vi "PLC.SendReasembly.vi"(8 "error in":errorcluster, 10 "Reasembly data":T11, 11 "Data_in":T1={"Status"={"Idx"=0, "ConnRef"=0, "State"=enum."Off", "LiveBitTimer"=timestamp(0 s since 1904-01-01)}, "Sets"={"Enable"=FALSE, "IP"="", "Rack"=0, "Slot"=0, "LifeBitTimer_s"=0.0, "DataBlockAddr_PCStatus"=0, "DataBlockAddr_PLCStatus"=1, "DataBlockAddr_PLCNewData"=[], "DataBlockSize_PLCNewData"=[], "DataBlockAddr_PLCChangeOver"=[], "DataBlockSize_PLCChangeOver"=[], "DataBlockAddr_PCChangeOver"=[], "DataBlockAddr_PLCCheckStatus"=[], "DataBlockSize_PLCCheckStatus"=[], "DataBlockAddr_PCCheckStatus"=[]}, "PCstatus"={"General"={"LifeBit"=FALSE, "DbRun"=FALSE}, "Stations"=[]}, "PLCstatus"={"General"={"LifeBit"=FALSE}, "Stations"=[]}}) -> (0 "error out":errorcluster, 2 "PlcConfirmation":T11, 3 "Data out":T1={"Status"={"Idx"=0, "ConnRef"=0, "State"=enum."Off", "LiveBitTimer"=timestamp(0 s since 1904-01-01)}, "Sets"={"Enable"=FALSE, "IP"="", "Rack"=0, "Slot"=0, "LifeBitTimer_s"=0.0, "DataBlockAddr_PCStatus"=0, "DataBlockAddr_PLCStatus"=1, "DataBlockAddr_PLCNewData"=[], "DataBlockSize_PLCNewData"=[], "DataBlockAddr_PLCChangeOver"=[], "DataBlockSize_PLCChangeOver"=[], "DataBlockAddr_PCChangeOver"=[], "DataBlockAddr_PLCCheckStatus"=[], "DataBlockSize_PLCCheckStatus"=[], "DataBlockAddr_PCCheckStatus"=[]}, "PCstatus"={"General"={"LifeBit"=FALSE, "DbRun"=FALSE}, "Stations"=[]}, "PLCstatus"={"General"={"LifeBit"=FALSE}, "Stations"=[]}})   [LabVIEW 2016]
uses:
  PLC.CheckStatusReassembly.ctl
  PLC.Data.ctl
  PLC.Data.Status.ctl
  PLC.State.ctl
  PLC.Data.Sets.ctl
  LowLevel/PLC.DataBlock.PCstatus.ctl
  LowLevel/PLC.DataBlock.PCstatus.General.ctl
  LowLevel/PLC.DataBlock.PCstatus.Station.ctl
  LowLevel/PLC.DataBlock.PLCstatus.ctl
  LowLevel/PLC.DataBlock.PLCstatus.General.ctl
  LowLevel/PLC.DataBlock.PLCstatus.Station.ctl
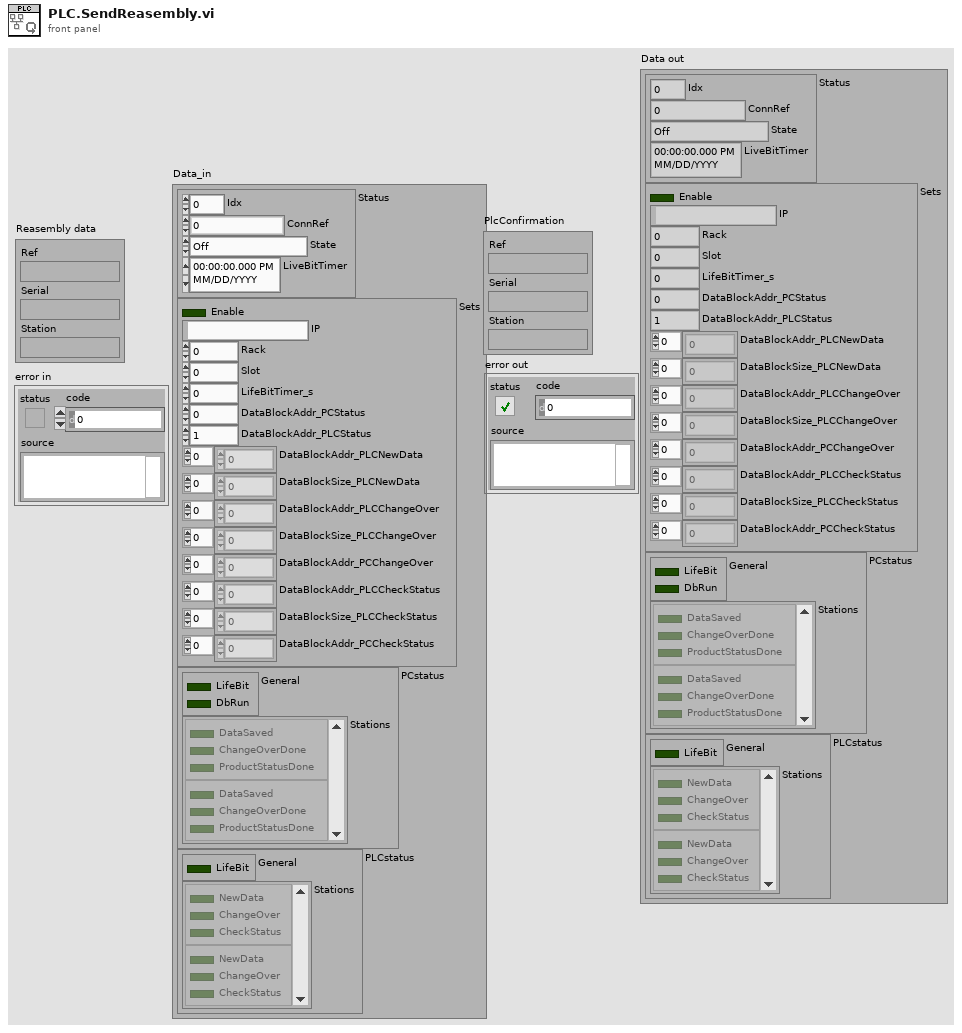
[diagram p1: front panel]
types:
  T1 = typedef "PLC.Data.ctl" = cluster{"Status":T2, "Sets":T4, "PCstatus":T5, "PLCstatus":T8}
  T2 = typedef "PLC.Data.Status.ctl" = cluster{"Idx":i32, "ConnRef":u64, "State":T3, "LiveBitTimer":timestamp}
  T3 = typedef "PLC.State.ctl" = enum32{"Off", "Error", "Idle", "Run"}
  T4 = typedef "PLC.Data.Sets.ctl" = cluster{"Enable":bool, "IP":string, "Rack":i32, "Slot":i32, "LifeBitTimer_s":dbl, "DataBlockAddr_PCStatus":i32, "DataBlockAddr_PLCStatus":i32, "DataBlockAddr_PLCNewData":i32[], "DataBlockSize_PLCNewData":i32[], "DataBlockAddr_PLCChangeOver":i32[], "DataBlockSize_PLCChangeOver":i32[], "DataBlockAddr_PCChangeOver":i32[], "DataBlockAddr_PLCCheckStatus":i32[], "DataBlockSize_PLCCheckStatus":i32[], "DataBlockAddr_PCCheckStatus":i32[]}
  T5 = typedef "PLC.DataBlock.PCstatus.ctl" = cluster{"General":T6, "Stations":T7[]}
  T6 = typedef "PLC.DataBlock.PCstatus.General.ctl" = cluster{"LifeBit":bool, "DbRun":bool}
  T7 = typedef "PLC.DataBlock.PCstatus.Station.ctl" = cluster{"DataSaved":bool, "ChangeOverDone":bool, "ProductStatusDone":bool}
  T8 = typedef "PLC.DataBlock.PLCstatus.ctl" = cluster{"General":T9, "Stations":T10[]}
  T9 = typedef "PLC.DataBlock.PLCstatus.General.ctl" = cluster{"LifeBit":bool}
  T10 = typedef "PLC.DataBlock.PLCstatus.Station.ctl" = cluster{"NewData":bool, "ChangeOver":bool, "CheckStatus":bool}
  T11 = typedef "PLC.CheckStatusReassembly.ctl" = cluster{"Ref":string, "Serial":string, "Station":string}
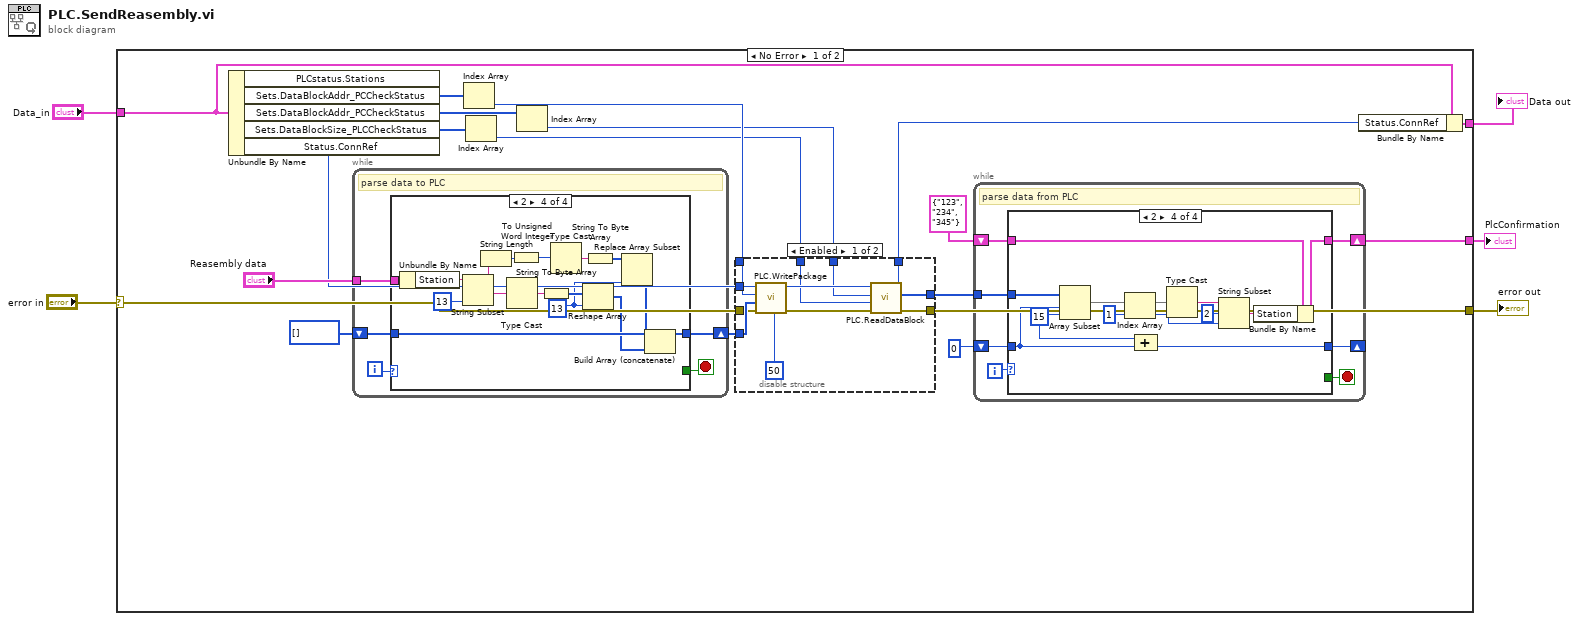
[diagram p0: block diagram]
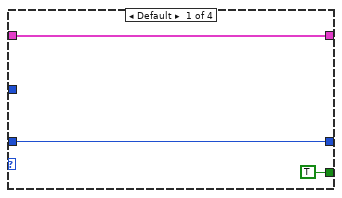
[diagram p3: hidden frame]
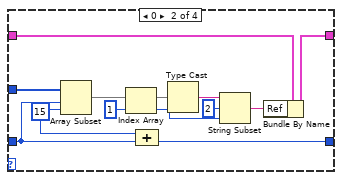
[diagram p4: hidden frame]
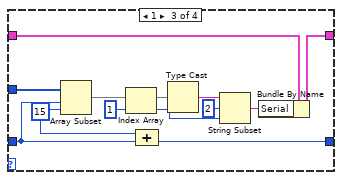
[diagram p5: hidden frame]
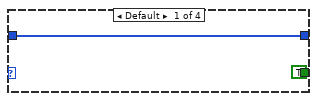
[diagram p6: hidden frame]
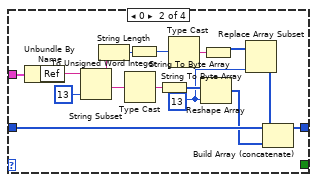
[diagram p7: hidden frame]
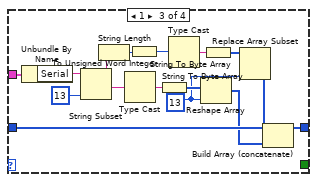
[diagram p8: hidden frame]
diagram:
  n1 = case shown="No Error" "error in" {
    selector: "error in" -> [w21 w137]
    tunnel: [w11 w137] -> w4
    tunnel: [w9 _] -> w3
    tunnel: "Data_in" -> [w8 w136]
    tunnel: [w6 w136] -> w1
    frame No Error {
      n2 = Unbundle By Name(w8) -> ("Sets.DataBlockAddr_PCCheckStatus"=w20:i32[], "Sets.DataBlockAddr_PCCheckStatus"=w17:i32[], "Sets.DataBlockSize_PLCCheckStatus"=w15:i32[], "Status.ConnRef"=w18:u64)  [unwired: 1 out]
      n3 = while {
        tunnel: "Reasembly data" -> [w87]
        shift-right: [w85] -> w23
        shift-left: u8[] [] ("data in") -> [w84]
        i -> [w88]
        stop <- w86 stop-if-true
        # "parse data to PLC"
        n4 = case shown="2" w88 {
          tunnel: w87 -> [_ w105 w110 w125]
          tunnel: [TRUE _ _ _] -> w86
          tunnel: [w89 w104 w120 w135] -> w85
          tunnel: w84 -> [w89 w103 w119 w134]
          frame Default {
          }
          frame 0 {
            w91 = 13 ("length (rest)")
            n5 = Unbundle By Name(w105) -> ("Ref"=w101:string)
            n6 = String Subset(string=w101, length (rest)=13 ("length (rest)")) -> (substring=w97:string)  [unwired: 1 in]
            n7 = String Length(string=w97) -> (length=w102:i32)
            n8 = Type Cast(x=w97) -> (*(type *) &x=w98:string)  [unwired: 1 in]
            n9 = To Unsigned Word Integer(number=w102) -> (unsigned 16bit integer=w100:u16)
            n10 = String To Byte Array(string=w98) -> (unsigned byte array=w96:u8[])
            n11 = Type Cast(x=w100) -> (*(type *) &x=w99:string)  [unwired: 1 in]
            n12 = Reshape Array(w96, w91) -> (w95:u8[])
            n13 = String To Byte Array(string=w99) -> (unsigned byte array=w93:u8[])
            n14 = Replace Array Subset(array=w93, new element=w91) -> (w92:u8[])  [unwired: 1 in]
            n15 = Build Array (concatenate)(w103, w92, w95) -> (w104:u8[])
          }
          frame 1 {
            w106 = 13 ("length (rest)")
            n16 = Unbundle By Name(w110) -> ("Serial"=w117:string)
            n17 = String Subset(string=w117, length (rest)=13 ("length (rest)")) -> (substring=w113:string)  [unwired: 1 in]
            n18 = String Length(string=w113) -> (length=w118:i32)
            n19 = Type Cast(x=w113) -> (*(type *) &x=w114:string)  [unwired: 1 in]
            n20 = To Unsigned Word Integer(number=w118) -> (unsigned 16bit integer=w116:u16)
            n21 = String To Byte Array(string=w114) -> (unsigned byte array=w112:u8[])
            n22 = Type Cast(x=w116) -> (*(type *) &x=w115:string)  [unwired: 1 in]
            n23 = Reshape Array(w112, w106) -> (w111:u8[])
            n24 = String To Byte Array(string=w115) -> (unsigned byte array=w109:u8[])
            n25 = Replace Array Subset(array=w109, new element=w106) -> (w107:u8[])  [unwired: 1 in]
            n26 = Build Array (concatenate)(w119, w107, w111) -> (w120:u8[])
          }
          frame 2 {
            w121 = 13 ("length (rest)")
            n27 = Unbundle By Name(w125) -> ("Station"=w132:string)
            n28 = String Subset(string=w132, length (rest)=13 ("length (rest)")) -> (substring=w128:string)  [unwired: 1 in]
            n29 = String Length(string=w128) -> (length=w133:i32)
            n30 = Type Cast(x=w128) -> (*(type *) &x=w129:string)  [unwired: 1 in]
            n31 = To Unsigned Word Integer(number=w133) -> (unsigned 16bit integer=w131:u16)
            n32 = String To Byte Array(string=w129) -> (unsigned byte array=w127:u8[])
            n33 = Type Cast(x=w131) -> (*(type *) &x=w130:string)  [unwired: 1 in]
            n34 = Reshape Array(w127, w121) -> (w126:u8[])
            n35 = String To Byte Array(string=w130) -> (unsigned byte array=w124:u8[])
            n36 = Replace Array Subset(array=w124, new element=w121) -> (w122:u8[])  [unwired: 1 in]
            n37 = Build Array (concatenate)(w134, w122, w126) -> (w135:u8[])
          }
        }
      }
      n38 = Index Array(array=w20) -> (element=w19:i32)  [unwired: 1 in]
      n39 = Index Array(array=w15) -> (element=w14:i32)  [unwired: 1 in]
      n40 = Index Array(array=w17) -> (element=w16:i32)  [unwired: 1 in]
      n41 = disable-structure shown="Enabled" {
        disable-tunnel: w23 -> [w35 w37]
        disable-tunnel: w21 -> [w34 _]
        disable-tunnel: w19 -> [w33 _]
        disable-tunnel: w18 -> [w32 _]
        disable-tunnel: w16 -> [w29 _]
        disable-tunnel: w14 -> [w28 _]
        disable-tunnel: [w27 w37] -> w12
        disable-tunnel: [w26 _] -> w11
        disable-tunnel: [w25 _] -> w7
        frame Enabled {
          n42 = call "PLC.WritePackage.vi"("max package size  (0: full)"=50, "error in (no error)"=w34, "data"=w35, "addr"=w33, "Ref in"=w32) -> ("error out"=w31:errorcluster, "Ref out"=w30:u64)  [unwired: 5 in]
          n43 = call "PLC.ReadDataBlock.vi"("error in (no error)"=w31, "Amount (1)"=w28, "Block"=w29, "Ref"=w30) -> ("error out"=w26:errorcluster, "data out"=w27:u8[], "ref out"=w25:u64)  [unwired: 5 in]
        }
        frame Disabled {
        }
      }
      n44 = while {
        tunnel: w12 -> [w39]
        shift-right: [w42] -> _
        shift-left: 0 -> [w43]
        shift-right: [w41] -> w9
        shift-left: T11 {"Ref"="123", "Serial"="234", "Station"="345"} ("Reasembly data 2") -> [w40]
        i -> [w44]
        stop <- w38 stop-if-true
        # "parse data from PLC"
        n45 = case shown="2" w44 {
          tunnel: w43 -> [w46 w50 w62 w74]
          tunnel: [w46 w49 w61 w73] -> w42
          tunnel: [w47 w59 w71 w83] -> w41
          tunnel: w40 -> [w47 w58 w70 w82]
          tunnel: w39 -> [_ w53 w65 w77]
          tunnel: [TRUE _ _ _] -> w38
          frame Default {
          }
          frame 0 {
            w51 = 15 ("length")
            n46 = Array Subset(array=w53, index=w50, length=w51) -> (w55:u8[])
            n47 = Index Array(array=w55, index=1) -> (element=w48:u8)
            n48 = Compound Arithmetic op=ADD(w51, w50) -> (w49:i32)
            n49 = Type Cast(x=w55) -> (*(type *) &x=w54:string)  [unwired: 1 in]
            n50 = String Subset(string=w54, offset (0)=2, length (rest)=w48) -> (substring=w52:string)
            n51 = Bundle By Name(cluster=w58, "Ref"=w52) -> (w59:T11)
          }
          frame 1 {
            w63 = 15 ("length")
            n52 = Array Subset(array=w65, index=w62, length=w63) -> (w67:u8[])
            n53 = Index Array(array=w67, index=1) -> (element=w60:u8)
            n54 = Compound Arithmetic op=ADD(w63, w62) -> (w61:i32)
            n55 = Type Cast(x=w67) -> (*(type *) &x=w66:string)  [unwired: 1 in]
            n56 = String Subset(string=w66, offset (0)=2, length (rest)=w60) -> (substring=w64:string)
            n57 = Bundle By Name(cluster=w70, "Serial"=w64) -> (w71:T11)
          }
          frame 2 {
            w75 = 15 ("length")
            n58 = Array Subset(array=w77, index=w74, length=w75) -> (w79:u8[])
            n59 = Index Array(array=w79, index=1) -> (element=w72:u8)
            n60 = Compound Arithmetic op=ADD(w75, w74) -> (w73:i32)
            n61 = Type Cast(x=w79) -> (*(type *) &x=w78:string)  [unwired: 1 in]
            n62 = String Subset(string=w78, offset (0)=2, length (rest)=w72) -> (substring=w76:string)
            n63 = Bundle By Name(cluster=w82, "Station"=w76) -> (w83:T11)
          }
        }
      }
      n64 = Bundle By Name(cluster=w8, "Status.ConnRef"=w7) -> (w6:T1)
    }
    frame Error {
    }
  }
  "error out" <- w4
  "Data out" <- w1
  "PlcConfirmation" <- w3
